vi "MouseMoved.vi"(8 "Error In":errorcluster, 10 "Coords":T1, 11 "reference in":refnum<class "Clippy.lvclass">) -> (0 "Error Out":errorcluster, 3 "reference out":refnum<class "Clippy.lvclass">)   [LabVIEW 2020, in "Clippy.lvclass"]
uses:
  Clippy.lvclass
  <vilib>/Utility/miscctls.llb/LVPoint32TypeDef.ctl
  AnimationTypes.ctl
  <vilib>/Analysis/coordinate.llb/Angle Range (Degree).ctl
  <vilib>/Analysis/coordinate.llb/Angle Units.ctl
  <vilib>/Analysis/coordinate.llb/Wrap Angle (scalar).vi
  <vilib>/Analysis/NI_AAL_Angle.lvlib
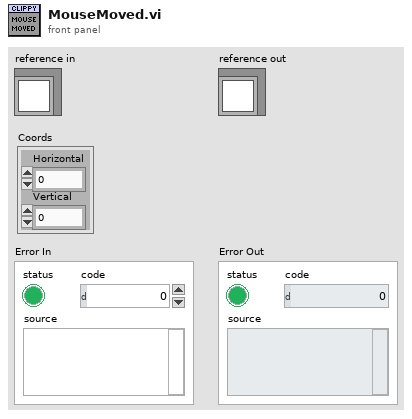
[diagram p1: front panel]
types:
  T1 = typedef "LVPoint32TypeDef.ctl" = cluster{"Horizontal":i32, "Vertical":i32}
  T2 = typedef "Clippy.lvclass/ObjectAttributes.ctl" = cluster{"ClippyPictureRef":refnum<vi>, "LastAnimation":T3, "LastAnimated":timestamp, "Visible":bool, "AnswerRef":refnum<vi>}
  T3 = typedef "Clippy.lvclass/AnimationTypes.ctl" = enum16{"Congratulate", "LookRight", "SendMail", "Thinking", "Explain", "IdleRopePile", "IdleAtom", "Print", "Hide", "GetAttention", "Save", "GetTechy", "GestureUp", "Idle1_1", "Processing", "Alert", "LookUpRight", "IdleSideToSide", "GoodBye", "LookLeft", "IdleHeadScratch", "LookUpLeft", "CheckingSomething", "Hearing_1", "GetWizardy", "IdleFingerTap", "GestureLeft", "Wave", "GestureRight", "Writing", "IdleSnooze", "LookDownRight", "GetArtsy", "Show", "LookDown", "Searching", "EmptyTrash", "Greeting", "LookUp", "GestureDown", "RestPose", "IdleEyeBrowRaise", "LookDownLeft"}
  T4 = typedef "NI_AAL_Angle.lvlib/Angle Units.ctl" = i32
  T5 = typedef "NI_AAL_Angle.lvlib/Angle Range (Degree).ctl" = u16
  T6 = typedef "LVPositionTypeDef.ctl" = cluster{"Left":i32, "Top":i32}
  T7 = typedef "LVBoundsTypeDef.ctl" = cluster{"Width":u32, "Height":u32}
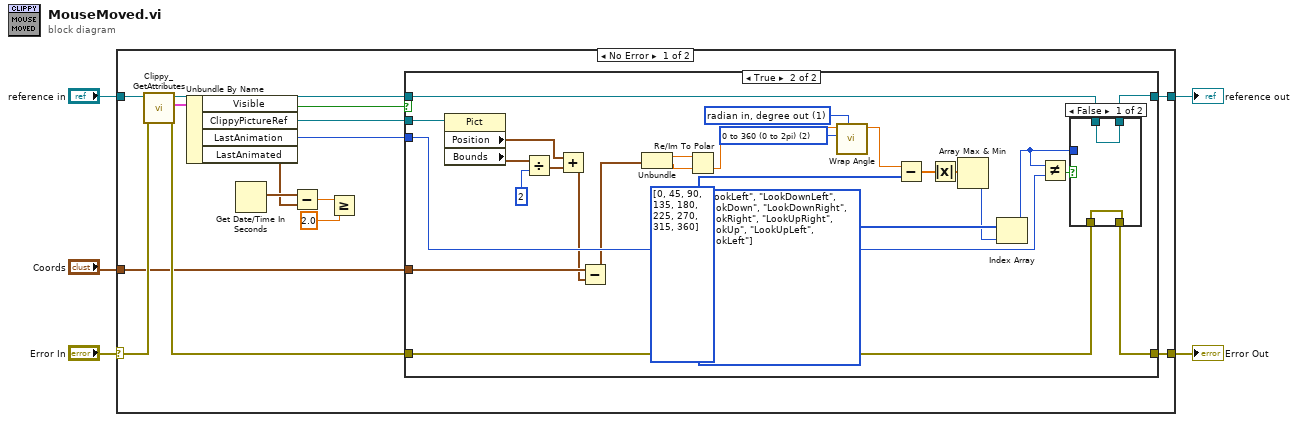
[diagram p0: block diagram]
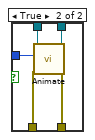
[diagram p3: hidden frame]
diagram:
  n1 = case shown="No Error" "Error In" {
    selector: "Error In" -> [w20 w57]
    tunnel: [w10 w57] -> w4
    tunnel: [w9 w56] -> w2
    tunnel: "reference in" -> [w18 w56]
    tunnel: "Coords" -> [w7 _]
    frame No Error {
      n2 = call "Clippy_GetAttributes.vi"("error in (no error)"=w20, "reference in"=w18) -> ("error out"=w11:errorcluster, "Data"=w19:T2, "reference out"=w8:refnum<class "Clippy.lvclass">)  [unwired: 6 in, 1 out]
      n3 = Unbundle By Name(w19) -> ("Visible"=w6:bool, "ClippyPictureRef"=w14:refnum<vi>, "LastAnimation"=w12:T3, "LastAnimated"=w16:timestamp)
      n4 = Get Date/Time In Seconds() -> (seconds since 1Jan1904=w17:timestamp)
      n5 = Subtract(x=w17, y=w16) -> (x-y=w15:dbl)
      n6 = Greater Or Equal?(x=w15, y=2.0) -> ()  [unwired: 1 out]
      n7 = case shown="True" w6 {
        tunnel: w14 -> [_ w48]
        tunnel: w12 -> [_ w41]
        tunnel: w8 -> [w22 w40]
        tunnel: w11 -> [w21 w39]
        tunnel: [w21 w38] -> w10
        tunnel: [w22 w37] -> w9
        tunnel: w7 -> [_ w25]
        frame False {
        }
        frame True {
          w34 = T4 1 items=["radian in, radian out", "radian in, degree out", "degree in, degree out", "degree in, radian out"] ("angle units")
          w35 = T5 2 items=["none", "-180 to 180 (-pi to pi)", "0 to 360 (0 to 2pi)"] ("angle range")
          w30 = T3[] [enum."LookLeft", enum."LookDownLeft", enum."LookDown", enum."LookDownRight", enum."LookRight", enum."LookUpRight", enum."LookUp", enum."LookUpLeft", enum."LookLeft"] items=["Congratulate", "LookRight", "SendMail", "Thinking", "Explain", "IdleRopePile", "IdleAtom", "Print", "Hide", "GetAttention", "Save", "GetTechy", "GestureUp", "Idle1_1", "Processing", "Alert", "LookUpRight", "IdleSideToSide", "GoodBye", "LookLeft", "IdleHeadScratch", "LookUpLeft", "CheckingSomething", "Hearing_1", "GetWizardy", "IdleFingerTap", "GestureLeft", "Wave", "GestureRight", "Writing", "IdleSnooze", "LookDownRight", "GetArtsy", "Show", "LookDown", "Searching", "EmptyTrash", "Greeting", "LookUp", "GestureDown", "RestPose", "IdleEyeBrowRaise", "LookDownLeft"] ("LastAnimation")
          n8 = property class="Pict"(reference=w48) -> ("Position"=w44:T6, "Bounds"=w47:T7)  [unwired: 1 in, 2 out]
          n9 = Divide(x=w47, y=2) -> (x/y=w45:cluster{"Width":dbl, "Height":dbl})
          n10 = Add(x=w44, y=w45) -> (x+y=w24:cluster{dbl, dbl})
          n11 = Subtract(x=w25, y=w24) -> (x-y=w23:cluster{dbl, dbl})
          n12 = Unbundle(w23) -> (w43:dbl, w42:dbl)
          n13 = Re/Im To Polar(2:w42, 3:w43) -> (0:w36:dbl)  [unwired: 1 out]
          n14 = call-poly <vilib>:"Wrap Angle.vi"("angle units"=w34, "angle range"=w35, "angle in"=w36) -> ("angle out"=w33:dbl)  [unwired: 7 in, 1 out]
          n15 = Subtract(x=w33, y=i32[] [0, 45, 90, 135, 180, 225, 270, 315, 360]) -> (x-y=w32:dbl[])
          n16 = Absolute Value(x=w32) -> (abs(x)=w31:dbl[])
          n17 = Array Max & Min(array=w31) -> (min index (indices)=w29:i32)  [unwired: 3 out]
          n18 = Index Array(array=w30, index=w29) -> (element=w28:T3)
          n19 = Not Equal?(x=w28, y=w41) -> (x != y?=w26:bool)
          n20 = case shown="False" w26 {
            tunnel: w40 -> [w49 w55]
            tunnel: w39 -> [w50 w54]
            tunnel: [w50 w53] -> w38
            tunnel: [w49 w52] -> w37
            tunnel: w28 -> [_ w51]
            frame False {
            }
            frame True {
              n21 = call-dynamic "Animate.vi"("Error In"=w54, "Animation"=w51, "reference in"=w55) -> ("Error Out"=w53:errorcluster, "reference out"=w52:refnum<class "Clippy.lvclass">)  [unwired: 7 in]
            }
          }
        }
      }
    }
    frame Error {
    }
  }
  "Error Out" <- w4
  "reference out" <- w2
